vi "Function of Time (SubVI).vi"(7 "N (rot)":u32, 8 "n":dbl, 11 "Final Angle":dbl) -> (0 "Total Time (s)":dbl, 2 "Next Angle":dbl, 3 "t (ms)":dbl, 4 "Current<=Final?":bool, 5 "dt (ms)":dbl)   [LabVIEW 2012]
uses:
  Function of Time Global.vi
  variables/GlobalUI.vi
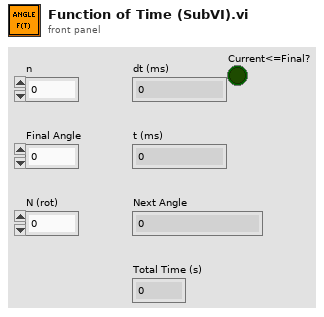
[diagram p1: front panel]
types:
  T1 = typedef "Stage Parameters.ctl" = cluster{"Scan Mode":T2, "Start position mm":dbl, "End position mm":dbl, "Velocity um/sec (continuous)":dbl, "Step size microns (discrete)":dbl, "Frames to grab (grab)":i32, "Sync Rotation with Stage":bool}
  T2 = typedef "ScanMode.ctl" = enum16{"None", "Continuous", "Point Scan (CH3 cursor)", "Point Scan Move (CH3 cursor)", "Grab", "Grab Move Stage", "Grab Move Z-stage", "Cont. Move Z-stage", "Spec Move Stage", "Spec Move Cont", "Surf Calib"}
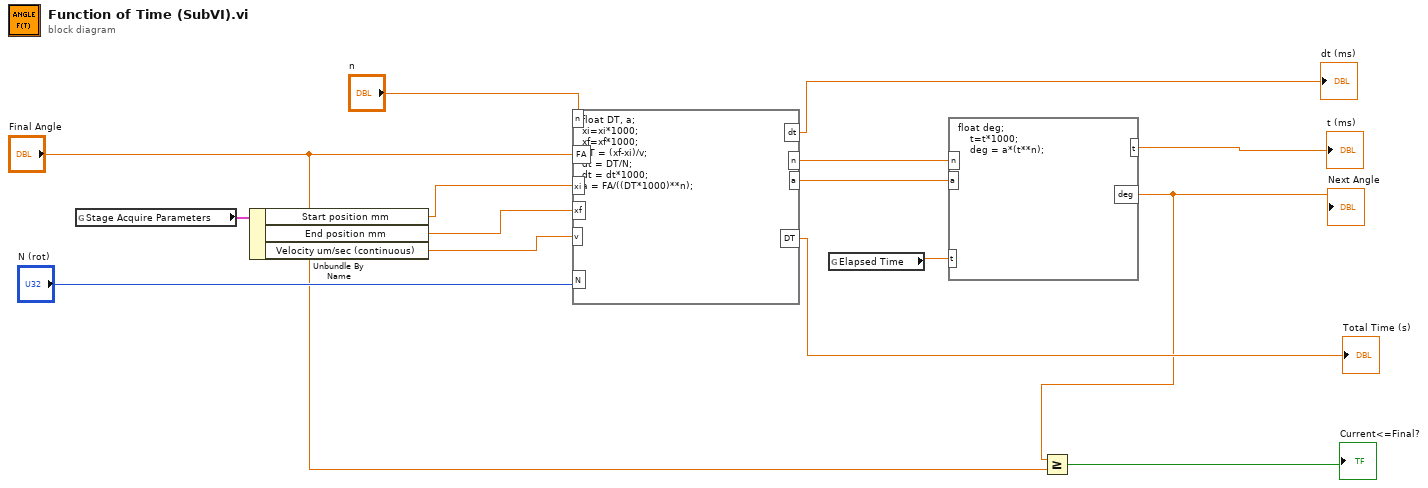
[diagram p0: block diagram]
diagram:
  n1 = global read "GlobalUI.vi" "Stage Acquire Parameters"() -> (w4:T1)
  n2 = Unbundle By Name(w4) -> ("Start position mm"=w3:dbl, "End position mm"=w2:dbl, "Velocity um/sec (continuous)"=w1:dbl)
  n3 = formula code="float DT, a;\nxi=xi*1000;\nxf=xf*1000;\nDT = (xf-xi)/v;\ndt = DT/N;\ndt = dt*1000;\na = FA/((DT*1000)**n);"("xi"=w3, "xf"=w2, "v"=w1, "N"="N (rot)", "FA"="Final Angle", "n"="n") -> ("dt"=→"dt (ms)":dbl, "DT"=→"Total Time (s)":dbl, "n"=w11:dbl, "a"=w12:dbl)
  n4 = global read "Function of Time Global.vi" "Elapsed Time"() -> (w8:dbl)
  n5 = formula code="float deg; \n    t=t*1000;\n    deg = a*(t**n);"("t"=w8, "n"=w11, "a"=w12) -> ("deg"=w6:dbl, "t"=→"t (ms)":dbl)
  "Next Angle" <- w6
  n6 = Greater Or Equal?(x=w6, y="Final Angle") -> (x >= y?=→"Current<=Final?":bool)
